vi "Concatenate.vi"(8 "error in (no error)":errorcluster, 10 "dataNpad":string, 11 "NPad2 in":refnum<class "NPad2.lvclass">) -> (0 "error out":errorcluster, 3 "NPad2 out":refnum<class "NPad2.lvclass">)   [LabVIEW 2020, in "NPad2.lvlib" / "NPad2.lvclass"]
uses:
  NPad2.lvclass
  NPad2.lvclass/NPad2.ctl
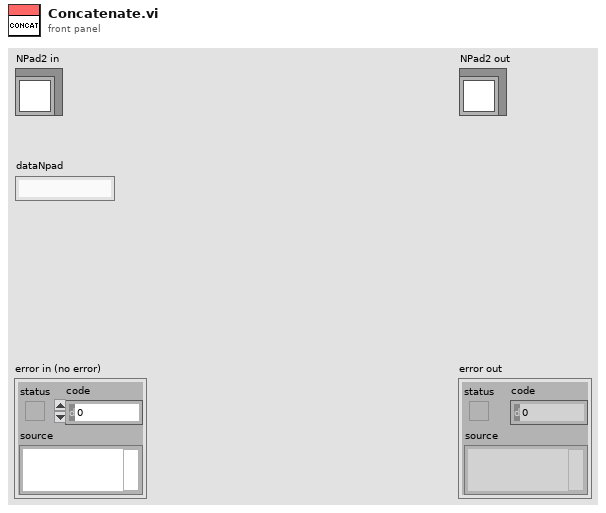
[diagram p1: front panel]
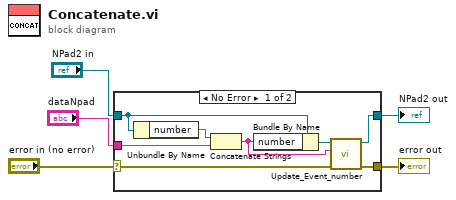
[diagram p0: block diagram]
diagram:
  n1 = case shown="No Error" "error in (no error)" {
    selector: "error in (no error)" -> [w7 w15]
    tunnel: [w6 w15] -> w4
    tunnel: [w13 w14] -> w2
    tunnel: "NPad2 in" -> [w10 w14]
    tunnel: "dataNpad" -> [w11 _]
    frame No Error {
      n2 = Unbundle By Name(w10) -> ("number"=w12:string)
      n3 = Concatenate Strings(w12, w11) -> (w8:string)
      n4 = Bundle By Name(cluster=w10, "number"=w8) -> (w9:refnum<class "NPad2.lvclass">)
      n5 = call "Update_Event_number.vi"("error in (no error)"=w7, "number"=w8, "NPad2 in"=w9) -> ("error out"=w6:errorcluster, "NPad2 out"=w13:refnum<class "NPad2.lvclass">)  [unwired: 7 in]
    }
    frame Error {
    }
  }
  "error out" <- w4
  "NPad2 out" <- w2
